vi "Switch Test Communications (7001).vi"(8 "error in (no error)":errorcluster, 11 "VISA resource name in":refnum<visa-resource-name>) -> (0 "error out":errorcluster, 3 "VISA resource name out":refnum<visa-resource-name>)   [LabVIEW 2016, in "Hall Effect Library.lvlib"]
uses:
  Hall Effect Library.lvlib
  <instrlib>/Keithley 7001/Keithley 7001.lvlib
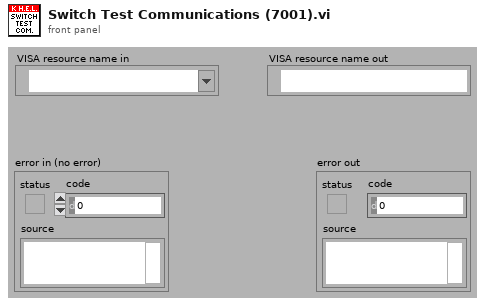
[diagram p1: front panel]
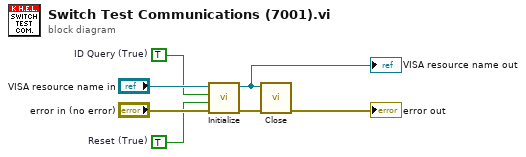
[diagram p0: block diagram]
diagram:
  w1 = TRUE  # Reset (True)
  w2 = TRUE  # ID Query (True)
  n1 = call <instrlib>:"Initialize.vi"("error in (no error)"="error in (no error)", "Reset (True)"=w1, "ID Query (True)"=w2, "VISA resource name"="VISA resource name in") -> ("error out"=w7:errorcluster, "VISA resource name out"=w5:refnum<visa-resource-name>)  [unwired: 1 in, 5 out]
  "VISA resource name out" <- w5
  n2 = call <instrlib>:"Close.vi"("error in (no error)"=w7, "VISA resource name"=w5) -> ("error out"=→"error out":errorcluster)  [unwired: 9 out]
